vi "Test Arduino VI Functionality.vi"() -> ()   [LabVIEW 2014]
uses:
  <vilib>/Aledyne-TSXperts/Arduino Compatible Compiler for LabVIEW/addons/Arduino MPU60X0/Arduino MPU60X0.lvlib
panel:
  out "number":i16
  in  "Boolean array":bool[](array[boolean])
  out "Boolean array correct one":bool[](array[boolean])
  in  "Numeric":i16
  out "Boolean array observed":bool[](array[boolean])
  out "Int":i16
  out "Error Out":errorcluster
  in  "Error In":errorcluster
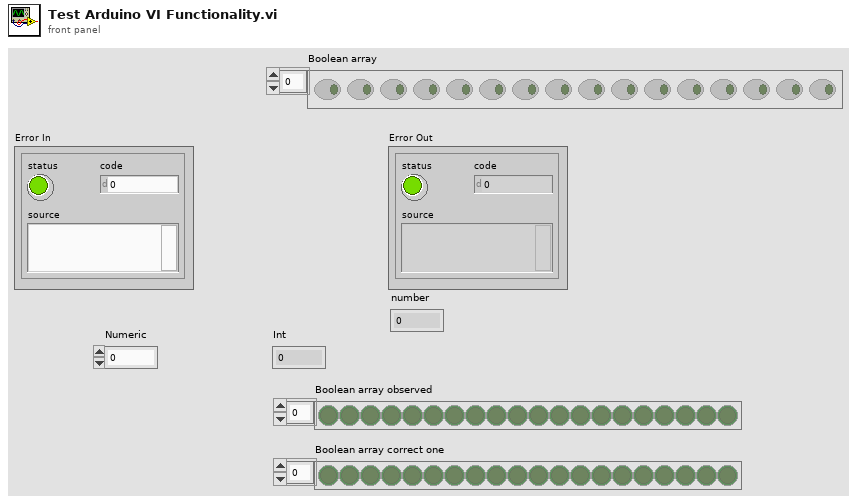
[diagram p1: front panel]
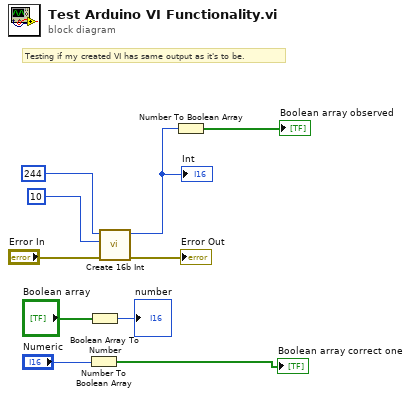
[diagram p0: block diagram]
diagram:
  # "Testing if my created VI has same output as it's to be."
  n1 = Number To Boolean Array(number="Numeric") -> (Boolean array=→"Boolean array correct one":bool[])
  n2 = Boolean Array To Number(Boolean array="Boolean array") -> (number=→"number":u32)
  n3 = call <vilib>:"Create 16b Int.vi"("Error In"="Error In", "LSB"=u8 10 ("MSB"), "MSB"=u8 244) -> ("Error Out"=→"Error Out":errorcluster, "Int"=w6:i16)  [unwired: 7 in]
  "Int" <- w6
  n4 = Number To Boolean Array(number=w6) -> (Boolean array=→"Boolean array observed":bool[])
